vi "MEMR-Preprocess Reanalysis.vi"(0 "Files":path[](array[path])=[path "D:/Data/MEMR/Ken/SFMH41-MEMR-1.txt", path "D:/Data/MEMR/Ken/SFMH41-MEMR-2.txt", path "D:/Data/MEMR/Ken/SFMH41-MEMR-3.txt"], 7 "Threshold":T1={"Measure"=enum."at max mag", "T(ms) re peak"=0.0, "Fmin (Hz)"=500.0, "Fmax (Hz)"=5000.0, "Window"=enum."None", "Resol (Hz)"=0.0, "Wpeak (Hz)"=0.0, "Criterion"=0.0, "Compute"=enum."Mean", "Scale"=enum."Linear"}, 9 "Force reanalyze":bool, 11 "Error In":errorcluster) -> (4 "preprocessed":T2, 8 "Threshold (from file)":T1, 10 "update threshold":bool, 15 "error out":errorcluster)   [LabVIEW 2020]
uses:
  MEMR-Offline Analysis Parameters.ctl
  MEMR-Processed Data.ctl
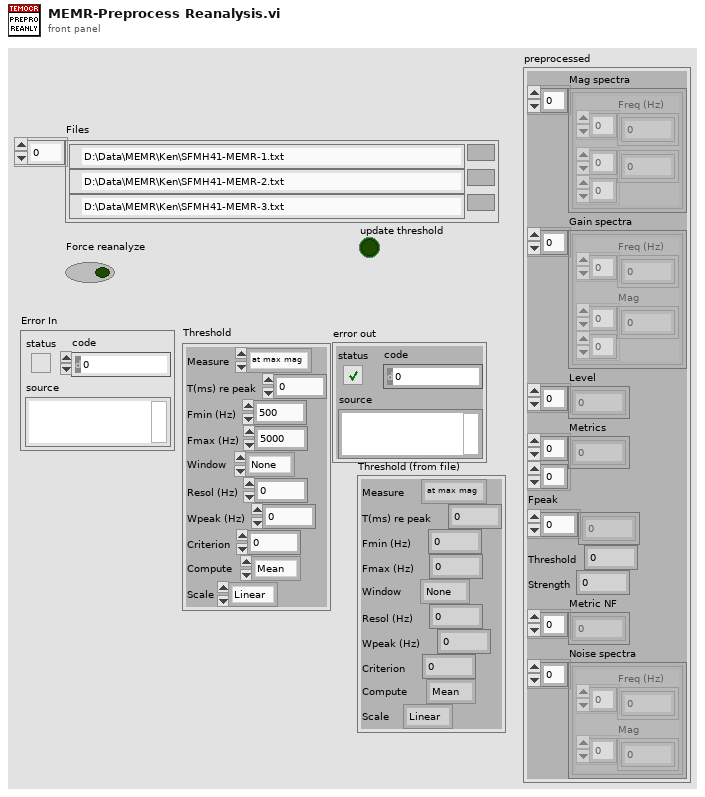
[diagram p1: front panel]
types:
  T1 = typedef "MEMR-Offline Analysis Parameters.ctl" = cluster{"Measure":enum16{"at max mag", "at max gain", "over window", "optimize", "Keefe"}, "T(ms) re peak":dbl, "Fmin (Hz)":dbl, "Fmax (Hz)":dbl, "Window":enum16{"None", "Hanning", "Hamming"}, "Resol (Hz)":dbl, "Wpeak (Hz)":dbl, "Criterion":dbl, "Compute":enum16{"Mean", "Sum"}, "Scale":enum16{"Linear", "Log"}}
  T2 = typedef "MEMR-Processed Data.ctl" = cluster{"Mag spectra":cluster{"Freq (Hz)":dbl[], dbl[][]}[], "Gain spectra":cluster{"Freq (Hz)":dbl[], "Mag":dbl[][]}[], "Level":dbl[], "Metrics":dbl[][], "Fpeak":dbl[], "Threshold":dbl, "Strength":dbl, "Metric NF":dbl[], "Noise spectra":cluster{"Freq (Hz)":dbl[], "Mag":dbl[]}[]}
  T3 = enum16{"open", "replace", "create", "open or create", "replace or create", "replace or create with confirmation"}
  T4 = cluster{"Measure":enum16{"at max mag", "at max gain", "over window", "optimize", "Keefe"}, "T(ms) re peak":dbl, "Fmin (Hz)":dbl, "Fmax (Hz)":dbl, "Window":enum16{"None", "Hanning", "Hamming"}, "Resol (Hz)":dbl, "Wpeak (Hz)":dbl, "Criterion":dbl, "Compute":enum16{"Mean", "Sum"}, "Scale":enum16{"Linear", "Log"}}
  T5 = typedef "MEMR-Params.ctl" = cluster{"Probe":T6, "Elicitor":T7, "Sequence":T9, "Analysis":T10, "Repeats":i32, "Timing":T11, "Save raw":bool, "Fs (Hz)":dbl}
  T6 = typedef "MEMR-Probe.ctl" = cluster{"Ear":enum16{"Right", "Left"}, "Stimulus":enum16{"Click", "Chirp"}, "Duration (us)":dbl, "Level":dbl}
  T7 = typedef "MEMR-Elicitor.ctl" = cluster{"Duration (ms)":dbl, "Ramp (ms)":dbl, "Transducer":T8}
  T8 = typedef "HSTS-Transducer.ctl" = enum16{"Insert", "TDH-39", "HD300", "ER-10X"}
  T9 = typedef "MEMR-Sequence.ctl" = cluster{"Start":dbl, "Stop":dbl, "Step":dbl}
  T10 = typedef "MEMR-Analysis.ctl" = cluster{"T(ms) re peak":dbl, "Fmin (Hz)":dbl, "Fmax (Hz)":dbl, "Window":enum16{"None", "Hanning", "Hamming"}, "Gain (dB)":dbl, "Resol (Hz)":dbl}
  T11 = typedef "MEMR-Timing.ctl" = cluster{"Click1-Noise (ms)":dbl, "Noise-Click2 (ms)":dbl, "ISI (ms)":dbl}
  T12 = typedef "MEMR-Analysis State.ctl" = cluster{"Data file":path, "Raw":refnum<file>, "PT":cluster{"Freq":dbl[], "Mag":dbl[]}, "IO":cluster{"Level":dbl[], "Mag":dbl[], "NF":dbl[]}, "Nreps":i32, "Fs (Hz)":dbl, "Sum":dbl[], "Nplot":i32, "Noff":i32, "Gain":dbl, "spectra":cluster{"Freq":dbl[], "Mag":dbl[][]}[], "gain":cluster{"Freq":dbl[], "Mag":dbl[]}[], "Baseline":dbl[]}
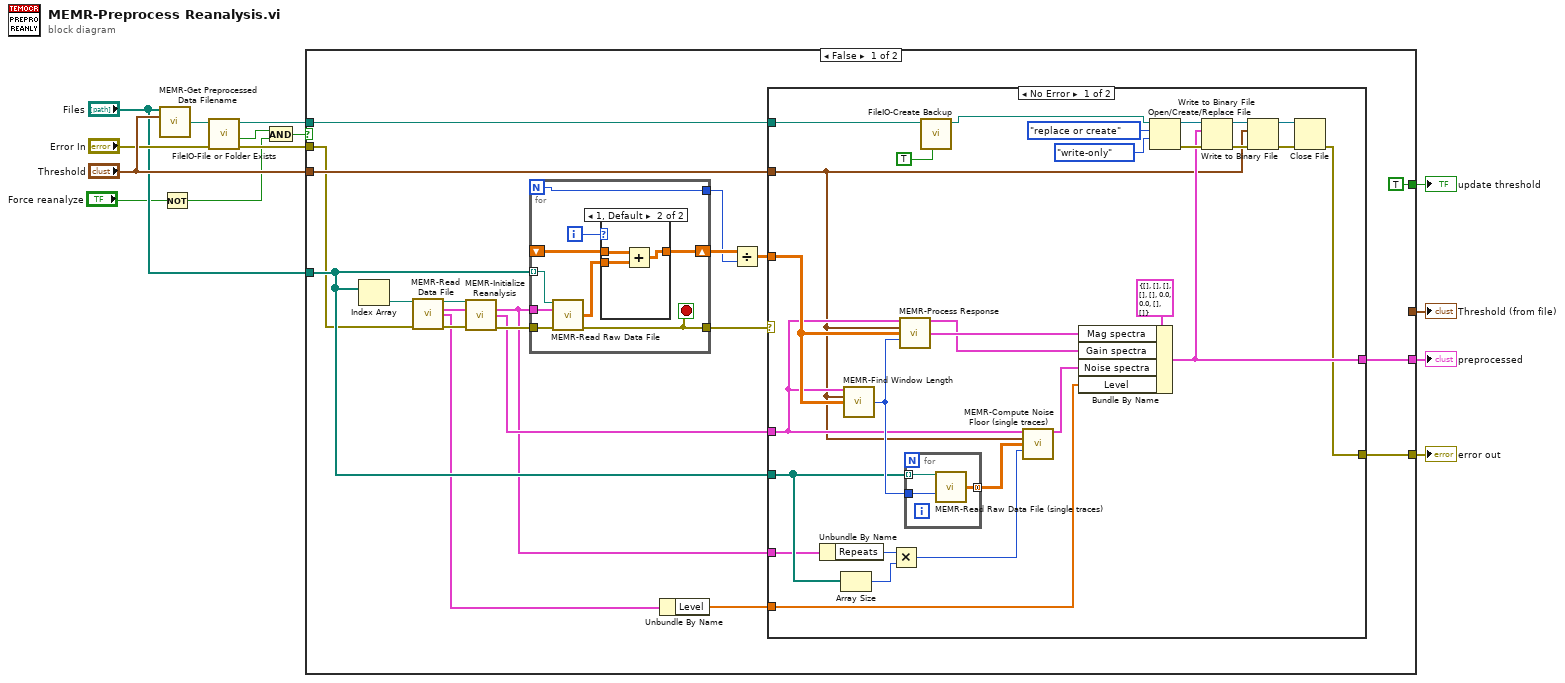
[diagram p0: block diagram]
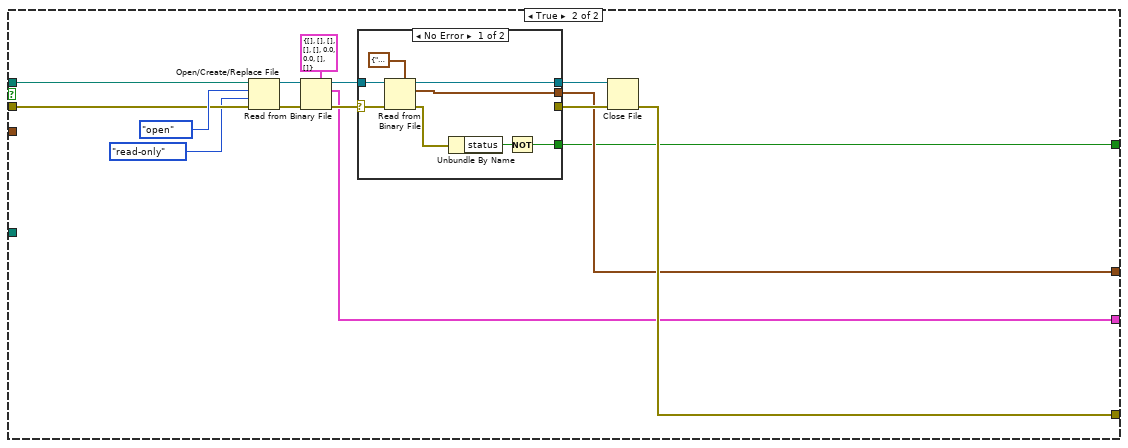
[diagram p4: hidden frame]
diagram:
  n1 = call "MEMR-Get Preprocessed Data Filename.vi"("Files"="Files", "Threshold"="Threshold") -> ("filename"=w11:path)  [unwired: 13 in]
  n2 = Not(x="Force reanalyze") -> (.not. x?=w3:bool)
  n3 = call "FileIO-File or Folder Exists.vi"("error in (no error)"="Error In", "path"=w11) -> ("error out"=w7:errorcluster, "Exists?"=w8:bool, "dup path"=w6:path)  [unwired: 6 in, 1 out]
  n4 = And(x=w8, y=w3) -> (x .and. y?=w4:bool)
  n5 = case shown="False" w4 {
    tunnel: [w26 w88] -> w14
    tunnel: [w25 w80] -> w13
    tunnel: "Threshold" -> [w24 _]
    tunnel: "Files" -> [w23 _]
    tunnel: w7 -> [w22 w90]
    tunnel: w6 -> [w21 w91]
    tunnel: [_ w82] -> w2
    tunnel: [TRUE w81] -> w1
    frame False {
      n6 = Index Array(array=w23) -> (element=w30:path)  [unwired: 1 in]
      n7 = call "MEMR-Read Data File.vi"("Path"=w30, "Error In"=w22) -> ("Path (dup)"=w34:path, "Params"=w19:T5, "IO"=w18:cluster{"Level":dbl[], "Gain":dbl[]}, "error out"=w33:errorcluster)  [unwired: 9 in, 1 out]
      n8 = call "MEMR-Initialize Reanalysis.vi"("Path"=w34, "Params"=w19, "error in"=w33) -> ("Params (dup)"=w16:T5, "State"=w20:T12, "error out"=w32:errorcluster)  [unwired: 9 in, 1 out]
      n9 = for {
        N -> [w68]
        tunnel: w16 -> [w74]
        tunnel: w32 -> [w75]
        tunnel: [w67] -> w31
        tunnel: w23 -> [w73] mode=indexing
        shift-right: [w70] -> w29
        shift-left: _ -> [w69]
        tunnel: [w68] -> w28
        i -> [w72]
        stop <- w67 stop-if-true
        n10 = call "MEMR-Read Raw Data File.vi"("Path"=w73, "Params"=w74, "error in"=w75) -> ("Array"=w71:dbl[][], "error out"=w67:errorcluster)  [unwired: 11 in]
        n11 = case shown="1, Default" w72 {
          tunnel: w71 -> [w76 w78]
          tunnel: [w76 w77] -> w70
          tunnel: w69 -> [_ w79]
          frame 0 {
          }
          frame 1, Default {
            n12 = Add(x=w79, y=w78) -> (x+y=w77:dbl[][])
          }
        }
      }
      n13 = Unbundle By Name(w18) -> ("Level"=w17:dbl[])
      n14 = Divide(x=w29, y=w28) -> (x/y=w27:dbl[][])
      n15 = case shown="No Error" w31 {
        selector: w31 -> [_ w66]
        tunnel: w20 -> [w56 _]
        tunnel: w24 -> [w35 _]
        tunnel: w27 -> [w62 _]
        tunnel: [w45 w66] -> w26
        tunnel: [w46 _] -> w25
        tunnel: w23 -> [w54 _]
        tunnel: w21 -> [w42 _]
        tunnel: w17 -> [w51 _]
        tunnel: w16 -> [w50 _]
        frame No Error {
          n16 = Unbundle By Name(w50) -> ("Repeats"=w55:i32)
          n17 = Array Size(array=w54) -> (size(s)=w53:i32)
          n18 = call "MEMR-Find Window Length.vi"("State In"=w56, "Analysis"=w35, "Avg"=w62) -> ("Window length"=w59:i32)  [unwired: 12 in]
          n19 = Multiply(x=w55, y=w53) -> (x*y=w49:i32)
          n20 = call "MEMR-Process Response.vi"("State In"=w56, "Analysis"=w35, "Avg"=w62, "Npts"=w59) -> ("Gain spectra"=w57:cluster{"Freq (Hz)":dbl[], "Mag":dbl[][]}[], "Mag spectra"=w60:cluster{"Freq (Hz)":dbl[], dbl[][]}[])  [unwired: 10 in]
          n21 = for {
            tunnel: w54 -> [w65] mode=indexing
            tunnel: [w64] -> w58 mode=concatenating
            tunnel: w59 -> [w63]
            n22 = call "MEMR-Read Raw Data File (single traces).vi"("Path"=w65, "length"=w63) -> ("Array"=w64:dbl[][])  [unwired: 12 in, 1 out]
          }
          n23 = call "FileIO-Create Backup.vi"("Append date"=TRUE, "Path"=w42) -> ("Path (thru)"=w41:path)  [unwired: 6 in, 3 out]
          n24 = call "MEMR-Compute Noise Floor (single traces).vi"("State In"=w56, "Analysis"=w35, "Avg"=w58, "Navg"=w49) -> ("Noise spectra"=w52:cluster{"Freq (Hz)":dbl[], "Mag (dB)":dbl[]}[])  [unwired: 11 in]
          n25 = Bundle By Name(cluster=T2 {"Mag spectra"=[], "Gain spectra"=[], "Level"=[], "Metrics"=[], "Fpeak"=[], "Threshold"=0.0, "Strength"=0.0, "Metric NF"=[], "Noise spectra"=[]} ("processed"), "Mag spectra"=w60, "Gain spectra"=w57, "Noise spectra"=w52, "Level"=w51) -> (w46:T2)
          n26 = Open/Create/Replace File(file path (use dialog)=w41, operation (0:open)=T3."replace or create", access (0:read/write)=enum16{"read/write", "read-only", "write-only"}."write-only") -> (refnum out=w47:refnum<file>, error out=w48:errorcluster)  [unwired: 3 in, 1 out]
          n27 = Write to Binary File(file (use dialog)=w47, data=w46, error in=w48) -> (refnum out=w39:refnum<file>, error out=w38:errorcluster)  [unwired: 3 in, 1 out]
          n28 = Write to Binary File(file (use dialog)=w39, data=w35, error in=w38) -> (refnum out=w37:refnum<file>, error out=w36:errorcluster)  [unwired: 3 in, 1 out]
          n29 = Close File(refnum=w37, error in=w36) -> (error out=w45:errorcluster)  [unwired: 1 out]
        }
        frame Error {
        }
      }
    }
    frame True {
      n30 = Open/Create/Replace File(file path (use dialog)=w91, error in=w90, operation (0:open)=T3."open", access (0:read/write)=enum16{"read/write", "read-only", "write-only"}."read-only") -> (refnum out=w93:refnum<file>, error out=w94:errorcluster)  [unwired: 2 in, 1 out]
      n31 = Read from Binary File(5:T2 {"Mag spectra"=[], "Gain spectra"=[], "Level"=[], "Metrics"=[], "Fpeak"=[], "Threshold"=0.0, "Strength"=0.0, "Metric NF"=[], "Noise spectra"=[]} ("processed"), 8:w94, 11:w93) -> (0:w86:errorcluster, 2:w80:T2, 3:w85:refnum<file>)  [unwired: 3 in, 1 out]
      n32 = case shown="No Error" w86 {
        selector: w86 -> [w102 w104]
        tunnel: w85 -> [w101 w103]
        tunnel: [_ w104] -> w84
        tunnel: [w100 w103] -> w83
        tunnel: [w99 _] -> w82
        tunnel: [w96 _] -> w81
        frame No Error {
          n33 = Read from Binary File(5:T4 {"Measure"=enum."at max mag", "T(ms) re peak"=0.0, "Fmin (Hz)"=0.0, "Fmax (Hz)"=0.0, "Window"=enum."None", "Resol (Hz)"=0.0, "Wpeak (Hz)"=0.0, "Criterion"=0.0, "Compute"=enum."Mean", "Scale"=enum."Linear"} ("Analysis"), 8:w102, 11:w101) -> (0:w97:errorcluster, 2:w99:T4, 3:w100:refnum<file>)  [unwired: 3 in, 1 out]
          n34 = Unbundle By Name(w97) -> ("status"=w98:bool)
          n35 = Not(x=w98) -> (.not. x?=w96:bool)
        }
        frame Error {
        }
      }
      n36 = Close File(refnum=w83, error in=w84) -> (error out=w88:errorcluster)  [unwired: 1 out]
    }
  }
  "error out" <- w14
  "preprocessed" <- w13
  "Threshold (from file)" <- w2
  "update threshold" <- w1
